vi "load.vi"(8 "error in (no error)":errorcluster, 10 "x/y/z path":path[](array[path]), 11 "PositionSignals in":refnum<class "PositionSignals.lvclass">) -> (0 "error out":errorcluster, 3 "PositionSignals out":refnum<class "PositionSignals.lvclass">)   [LabVIEW 2010, in "PositionSignals.lvclass"]
uses:
  PositionSignals.lvclass
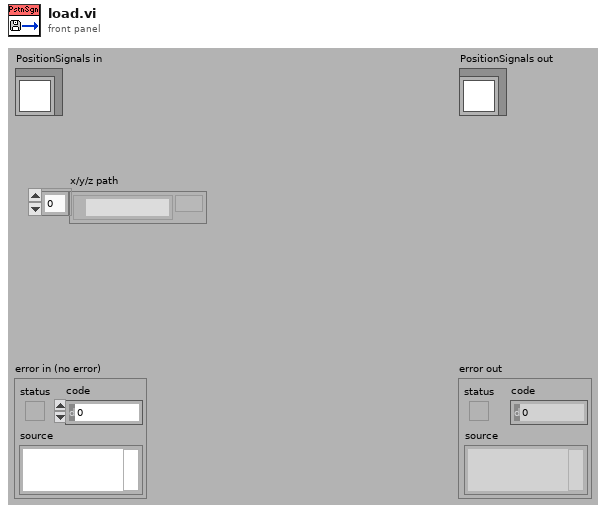
[diagram p1: front panel]
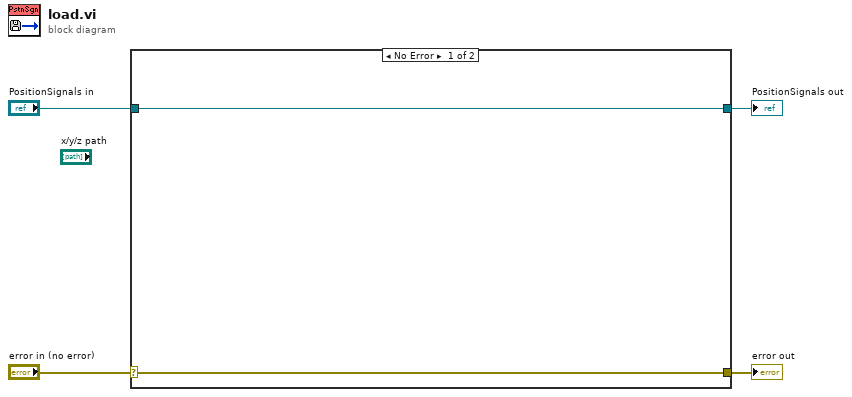
[diagram p0: block diagram]
diagram:
  n1 = case shown="No Error" "error in (no error)" {
    selector: "error in (no error)" -> [w5 w8]
    tunnel: [w5 w8] -> w3
    tunnel: [w6 w7] -> w1
    tunnel: "PositionSignals in" -> [w6 w7]
    frame No Error {
    }
    frame Error {
    }
  }
  "error out" <- w3
  "PositionSignals out" <- w1
